vi "FringeTrackerController.vi"() -> ()   [LabVIEW 2009]
uses:
  Controls/FringeTrackerState.ctl
  Controls/FringeTrackerInfo.ctl
  Nicmos/Controls/NICMOS.READOUT.ctl
  Controls/FringTrackerCommand.ctl
  Controls/FringeTrackerData.ctl
panel:
  out "FringeTrackerInfo":T1={"Readout"={"Readout"=100, "Deglitch"=10, "Framerate"=200.0, "Bank"=2}, "OPD stroke"=0.0, "OPD per pixel"=0.0}
  out "Wavelength":dbl[unit]
  out "State":T3
  in  "PROCESS":string="FRINGETRACKER"
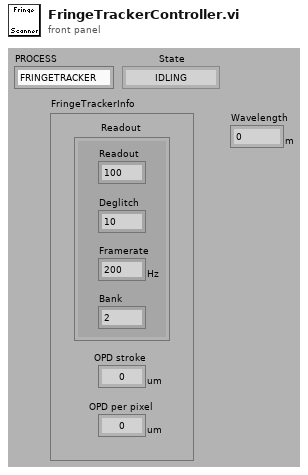
[diagram p1: front panel]
types:
  T1 = typedef "FringeTrackerInfo.ctl" = cluster{"Readout":T2, "OPD stroke":dbl[unit], "OPD per pixel":dbl[unit]}
  T2 = typedef "NICMOS.READOUT.ctl" = cluster{"Readout":i32, "Deglitch":i32, "Framerate":dbl[unit], "Bank":i32}
  T3 = typedef "FringeTrackerState.ctl" = enum16{"IDLING", "CONFIGURING", "SCANNING", "SEARCHING", "TRACKING", "STOPPING"}
  T4 = typedef "FringeTrackerData.ctl" = cluster{"Readout":T2, "Wavelength":dbl[unit], "Frame per fringe":dbl, "Autcollimation":bool, "OPD stroke":dbl[unit], "OPD per pixel":dbl[unit], "Offset":dbl[unit]}
  T5 = typedef "FringTrackerCommand.ctl" = cluster{"Command":enum16{"IDLE", "SCAN", "TRACK", "QUIT"}, "FringeTrackerData":T4}
  T6 = typedef "FringeTrackerSynchro.ctl" = cluster{"Command":refnum<queue>, "State":refnum<notifier>, "Info":refnum<notifier>, "NicmosData":refnum<notifier>}
  T7 = typedef "PIEZO.WAVE.ctl" = cluster{"Speed":dbl[unit], "Stiffness (0.95)":dbl, "Linear Stroke":dbl[unit], "Delay":dbl[unit]}
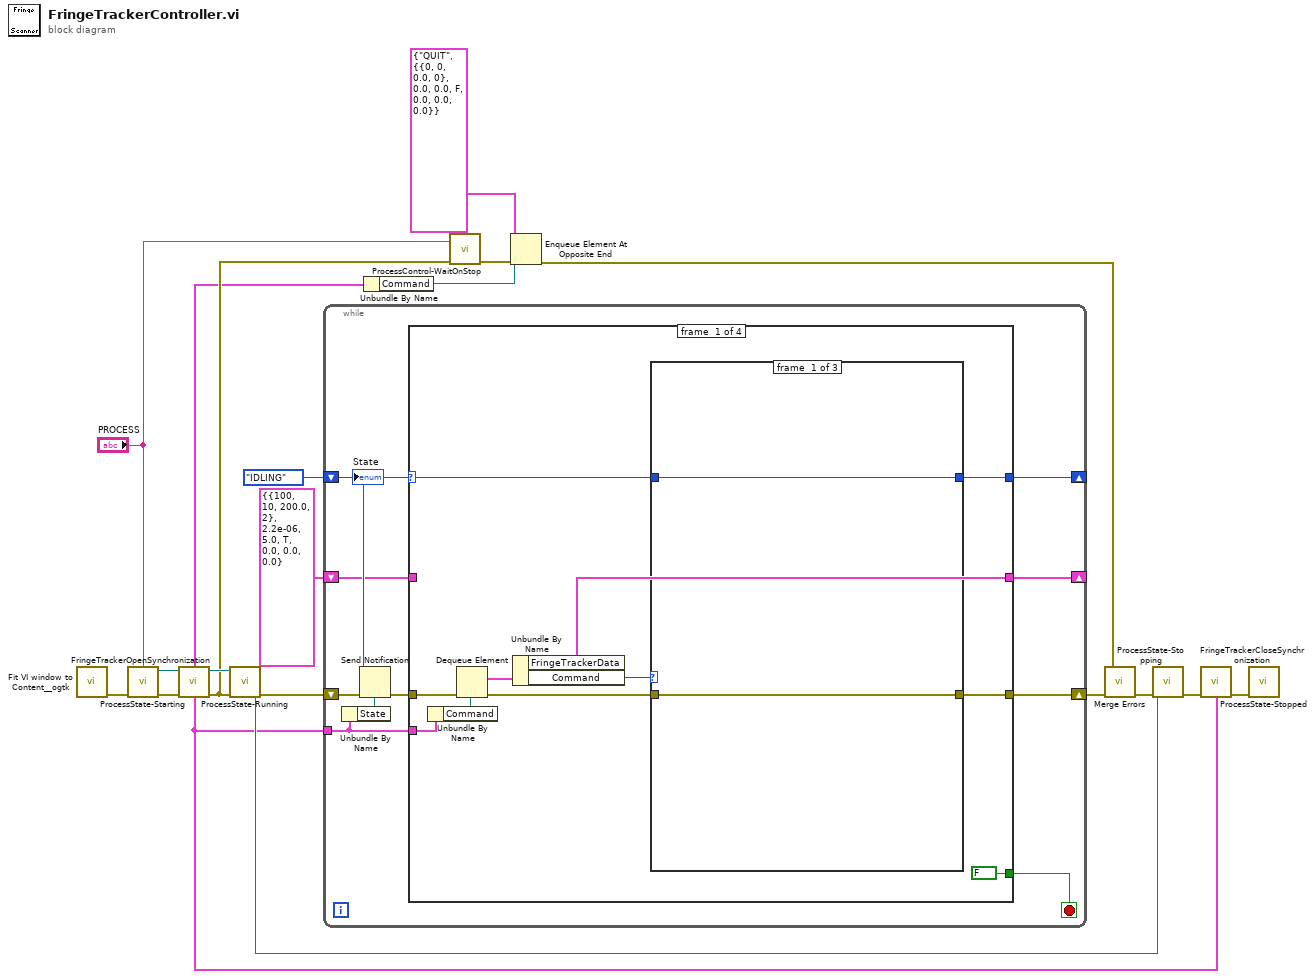
[diagram p0: block diagram]
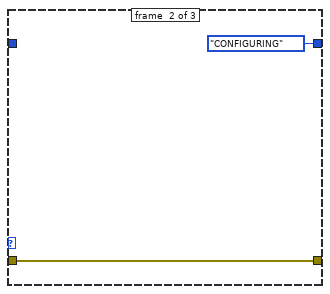
[diagram p2: hidden frame]
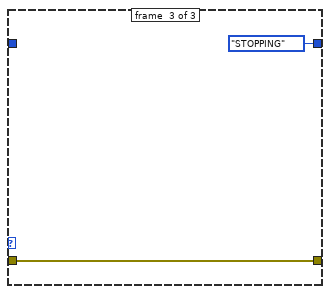
[diagram p3: hidden frame]
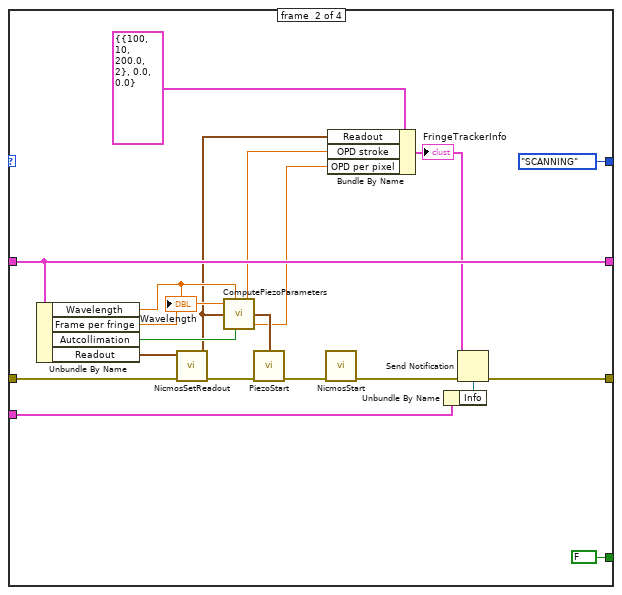
[diagram p4: hidden frame]
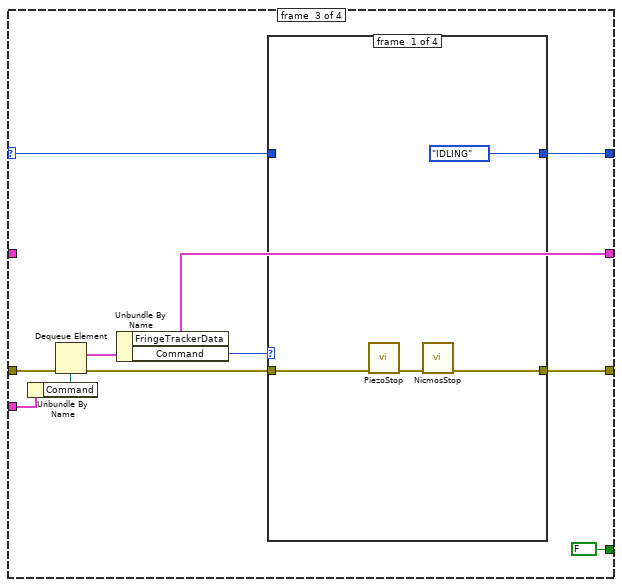
[diagram p5: hidden frame]
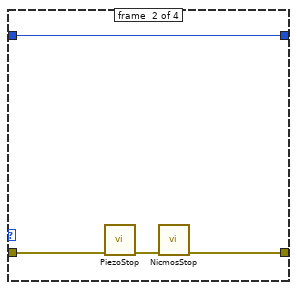
[diagram p6: hidden frame]
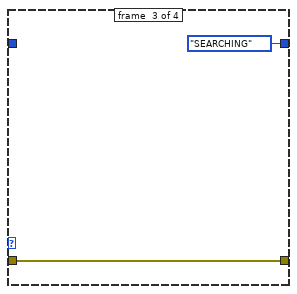
[diagram p7: hidden frame]
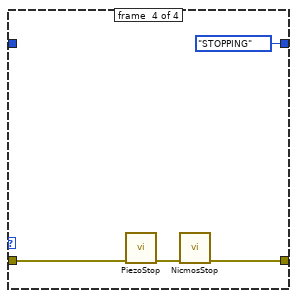
[diagram p8: hidden frame]
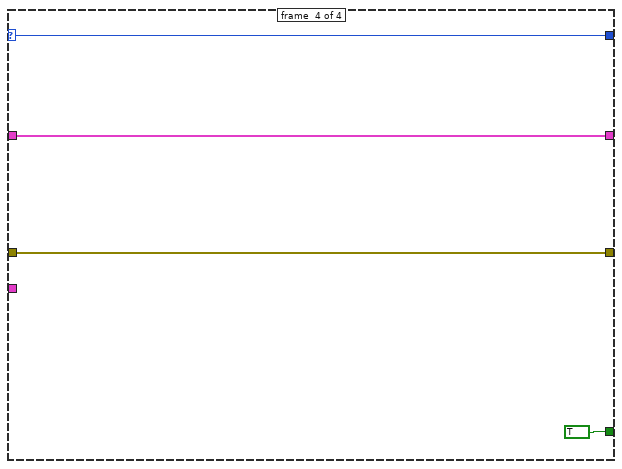
[diagram p9: hidden frame]
diagram:
  n1 = call <userlib>:"Fit VI window to Content__ogtk.vi"() -> ("error out"=w18:errorcluster)  [unwired: 6 in, 1 out]
  n2 = call "ProcessState-Starting.vi"("PROCESS"="PROCESS", "error in (no error)"=w18) -> ("ProcessStateNotifier"=w14:refnum<notifier>, "error in (no error)"=w16:errorcluster)  [unwired: 6 in]
  n3 = call "FringeTrackerOpenSynchronization.vi"("error in (no error)"=w16) -> ("FringeTrackerSynchro"=w2:T6, "error out"=w13:errorcluster)  [unwired: 7 in]
  n4 = call "ProcessState-Running.vi"("ProcessStateNotifier in"=w14, "error in (no error)"=w13) -> ("ProcessStateNotifier out"=w5:refnum<notifier>, "error out"=w15:errorcluster)  [unwired: 6 in]
  n5 = while {
    shift-right: [w23] -> w8
    shift-left: w15 -> [w28]
    shift-right: [w22] -> _
    shift-left: FringeTrackerState."IDLING" ("FringeTrackerState") -> [w25]
    tunnel: w2 -> [w24]
    shift-right: [w20] -> _
    shift-left: T4 {"Readout"={"Readout"=100, "Deglitch"=10, "Framerate"=200.0, "Bank"=2}, "Wavelength"=2.2e-06, "Frame per fringe"=5.0, "Autcollimation"=TRUE, "OPD stroke"=0.0, "OPD per pixel"=0.0, "Offset"=0.0} ("FringeTrackerData") -> [w19]
    stop <- w21 stop-if-true
    n6 = Unbundle By Name(w24) -> ("State"=w26:refnum<notifier>)
    n7 = Send Notification(notification=w25, notifier=w26, error in (no error)=w28) -> (error out=w27:errorcluster)  [unwired: 1 out]
    n8 = case shown="\"SCANNING\"" w25 {
      selector: w25 -> [w34 _ w71 w94]
      tunnel: w27 -> [w38 w62 w75 w93]
      tunnel: w24 -> [w39 w50 w76 _]
      tunnel: [w35 w48 w72 w93] -> w23
      tunnel: [w33 FringeTrackerState."SCANNING" ("FringeTrackerState") w70 w94] -> w22
      tunnel: [FALSE FALSE FALSE TRUE] -> w21
      tunnel: [w29 w55 w66 w91] -> w20
      tunnel: w19 -> [_ w55 _ w91]
      frame #0 {
        n9 = Unbundle By Name(w39) -> ("Command"=w37:refnum<queue>)
        n10 = Dequeue Element(queue=w37, error in (no error)=w38) -> (element=w30:T5, error out=w36:errorcluster)  [unwired: 1 in, 2 out]
        n11 = Unbundle By Name(w30) -> ("FringeTrackerData"=w29:T4, "Command"=w31:enum16{"IDLE", "SCAN", "TRACK", "QUIT"})
        n12 = case shown="\"IDLE\", Default" w31 {
          tunnel: w36 -> [w41 w42 w44]
          tunnel: [w41 w42 w44] -> w35
          tunnel: w34 -> [w40 _ _]
          tunnel: [w40 FringeTrackerState."CONFIGURING" ("FringeTrackerState") FringeTrackerState."STOPPING" ("FringeTrackerState")] -> w33
          frame #0 {
          }
          frame #1 {
          }
          frame #2 {
          }
        }
      }
      frame #1 {
        n13 = Unbundle By Name(w55) -> ("Wavelength"=w56:dbl[unit], "Frame per fringe"=w57:dbl, "Autcollimation"=w58:bool, "Readout"=w59:T2)
        "Wavelength" <- w56
        n14 = call "NicmosSetReadout.vi"("READOUT in"=w59, "error in (no error)"=w62) -> ("READOUT out"=w53:T2, "error out"=w65:errorcluster)  [unwired: 6 in]
        n15 = call "ComputePiezoParameters.vi"("Frame per fringe"=w57, "Wavelength"=w56, "READOUT"=w53, "Autcollimation"=w58) -> ("OPD stroke"=w52:dbl[unit], "WAVE"=w63:T7, "OPD per pixel"=w51:dbl[unit])  [unwired: 1 in]
        n16 = call "PiezoStart.vi"("WAVE"=w63, "error in (no error)"=w65) -> ("error out"=w64:errorcluster)  [unwired: 7 in]
        n17 = call "NicmosStart.vi"("error in (no error)"=w64) -> ("error out"=w49:errorcluster)  [unwired: 8 in]
        n18 = Bundle By Name(cluster=T1 {"Readout"={"Readout"=100, "Deglitch"=10, "Framerate"=200.0, "Bank"=2}, "OPD stroke"=0.0, "OPD per pixel"=0.0} ("FringeTrackerInfo"), "Readout"=w53, "OPD stroke"=w52, "OPD per pixel"=w51) -> (w46:T1)
        "FringeTrackerInfo" <- w46
        n19 = Unbundle By Name(w50) -> ("Info"=w47:refnum<notifier>)
        n20 = Send Notification(notification=w46, notifier=w47, error in (no error)=w49) -> (error out=w48:errorcluster)  [unwired: 1 out]
      }
      frame #2 {
        n21 = Unbundle By Name(w76) -> ("Command"=w74:refnum<queue>)
        n22 = Dequeue Element(queue=w74, error in (no error)=w75) -> (element=w67:T5, error out=w73:errorcluster)  [unwired: 1 in, 2 out]
        n23 = Unbundle By Name(w67) -> ("FringeTrackerData"=w66:T4, "Command"=w68:enum16{"IDLE", "SCAN", "TRACK", "QUIT"})
        n24 = case shown="\"SCAN\"" w68 {
          tunnel: w73 -> [w80 w83 w85 w89]
          tunnel: [w78 w82 w85 w88] -> w72
          tunnel: w71 -> [_ w81 _ _]
          tunnel: [FringeTrackerState."IDLING" ("FringeTrackerState") w81 FringeTrackerState."SEARCHING" ("FringeTrackerState") FringeTrackerState."STOPPING" ("FringeTrackerState")] -> w70
          frame #0 {
            n25 = call "PiezoStop.vi"("error in (no error)"=w80) -> ("error out"=w79:errorcluster)  [unwired: 10 in]
            n26 = call "NicmosStop.vi"("error in (no error)"=w79) -> ("error out"=w78:errorcluster)  [unwired: 8 in]
          }
          frame #1 {
            n27 = call "PiezoStop.vi"("error in (no error)"=w83) -> ("error out"=w84:errorcluster)  [unwired: 10 in]
            n28 = call "NicmosStop.vi"("error in (no error)"=w84) -> ("error out"=w82:errorcluster)  [unwired: 8 in]
          }
          frame #2 {
          }
          frame #3 {
            n29 = call "PiezoStop.vi"("error in (no error)"=w89) -> ("error out"=w90:errorcluster)  [unwired: 10 in]
            n30 = call "NicmosStop.vi"("error in (no error)"=w90) -> ("error out"=w88:errorcluster)  [unwired: 8 in]
          }
        }
      }
      frame #3 {
      }
    }
    "State" <- w25
  }
  n31 = Unbundle By Name(w2) -> ("Command"=w10:refnum<queue>)
  n32 = call "ProcessControl-WaitOnStop.vi"("PROCESS"="PROCESS", "error out"=w13) -> ("error in"=w11:errorcluster)  [unwired: 7 in]
  n33 = Enqueue Element At Opposite End(queue=w10, element=T5 {"Command"=enum."QUIT", "FringeTrackerData"={"Readout"={"Readout"=0, "Deglitch"=0, "Framerate"=0.0, "Bank"=0}, "Wavelength"=0.0, "Frame per fringe"=0.0, "Autcollimation"=FALSE, "OPD stroke"=0.0, "OPD per pixel"=0.0, "Offset"=0.0}} ("FringeTrackerCommand"), error in (no error)=w11) -> (error out=w7:errorcluster)  [unwired: 1 in, 2 out]
  n34 = call <vilib>:"Merge Errors.vi"("error in 3 (no error)"=w8, "error in 1 (no error)"=w7) -> ("error out"=w6:errorcluster)  [unwired: 5 in]
  n35 = call "ProcessState-Stopping.vi"("ProcessStateNotifier in"=w5, "error in (no error)"=w6) -> ("error out"=w4:errorcluster)  [unwired: 6 in, 1 out]
  n36 = call "FringeTrackerCloseSynchronization.vi"("FringeTrackerSynchro"=w2, "error in (no error)"=w4) -> ("error out"=w3:errorcluster)  [unwired: 7 in]
  n37 = call "ProcessState-Stopped.vi"("error in (no error)"=w3) -> ()  [unwired: 8 in, 1 out]
